vi "3_1.vi"() -> ()   [LabVIEW 2010]
panel:
  in  "stop":bool
  in  "OK Button":bool
  out "appended array":bool[](array[boolean])
  in  "7":bool
  in  "8":bool
  in  "6":bool
  in  "9":bool
  in  "10":bool
  in  "5":bool
  in  "4":bool
  in  "1":bool
  in  "3":bool
  in  "2":bool
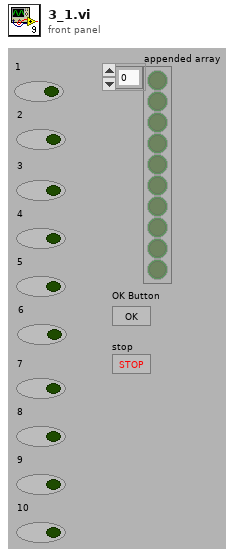
[diagram p1: front panel]
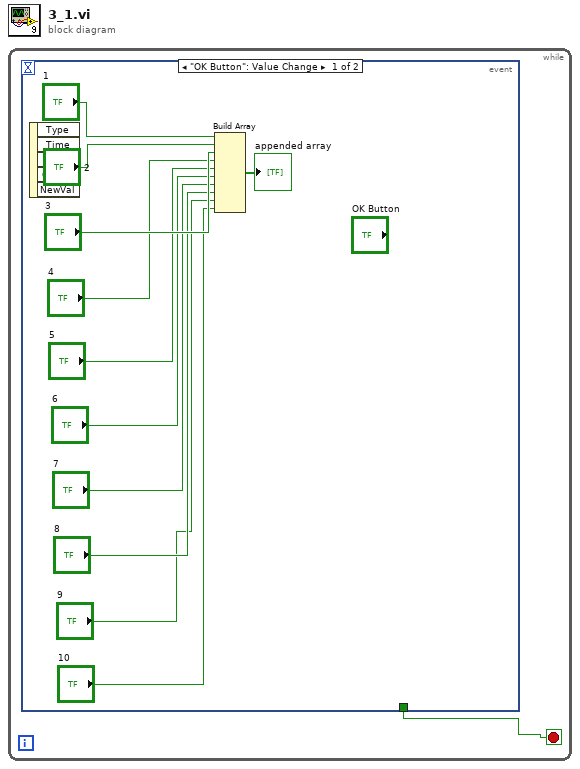
[diagram p0: block diagram]
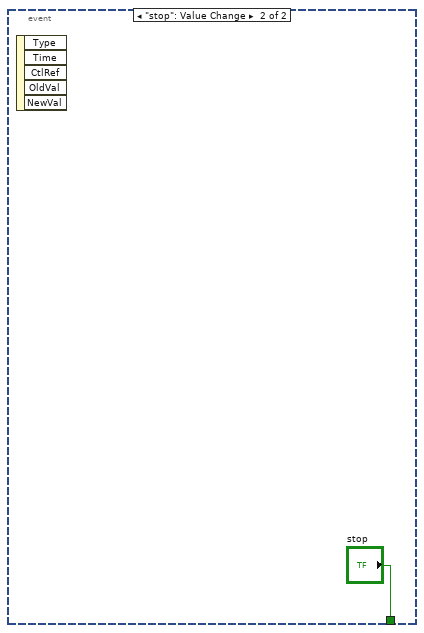
[diagram p2: hidden frame]
diagram:
  n1 = while {
    stop <- w1 stop-if-true
    n2 = event shown="[0] \"OK Button\": Value Change" {
      selector: _ -> [_ _]
      dyn-events: _ -> [_ _]
      timeout: _ -> [_ _]
      tunnel: [_ "stop"] -> w1
      event "OK Button": Value Change {
        n3 = event-data() -> ()  [unwired: 1 in, 5 out]
        n4 = Build Array("1", "2", "3", "4", "5", "6", "7", "8", "9", "10") -> (→"appended array":bool[])
      }
      event "stop": Value Change {
        n5 = event-data() -> ()  [unwired: 1 in, 5 out]
      }
    }
  }
